vi "DereferencingPointerToInteger.vi"(8 "error in (no error)":errorcluster, 11 "Address (Pointer)":i64) -> (0 "error out":errorcluster, 3 "Value":i32)   [LabVIEW 2009, in "LabVIEWWrapper_PassingDataSampleDLL.lvlib"]
uses:
  LabVIEWWrapper_PassingDataSampleDLL.lvlib
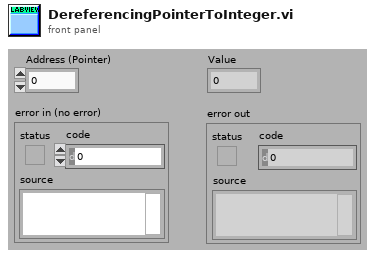
[diagram p1: front panel]
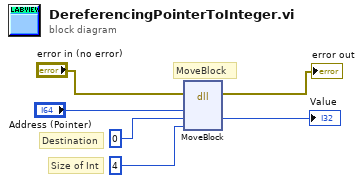
[diagram p0: block diagram]
diagram:
  # "Destination"
  # "Size of Int"
  # "MoveBlock"
  n1 = dll-call lib="LabVIEW" fn="MoveBlock"(error in="error in (no error)", "Address (Pointer)"="Address (Pointer)", "Destination"=0, "Size"=4 ("arg3")) -> (error out=→"error out":errorcluster, "Destination"=→"Value":i32)  [unwired: 5 in, 1 out]
